vi "getSetting.vi"(8 "error in":errorcluster, 9 "Parameter":string="estimator_strategy", 10 "Array Parameter List":string[](array[string])=["izn3", "icomp"], 11 "Path":path=path "/home/ttsai/Documents/stash/ts_tcs_ofc/configData/pinv.esti") -> (0 "error out":errorcluster, 1 "Value":string)   [LabVIEW 2016]
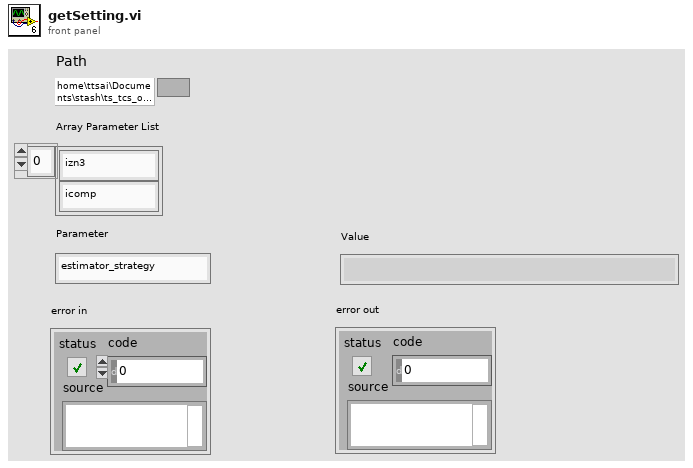
[diagram p1: front panel]
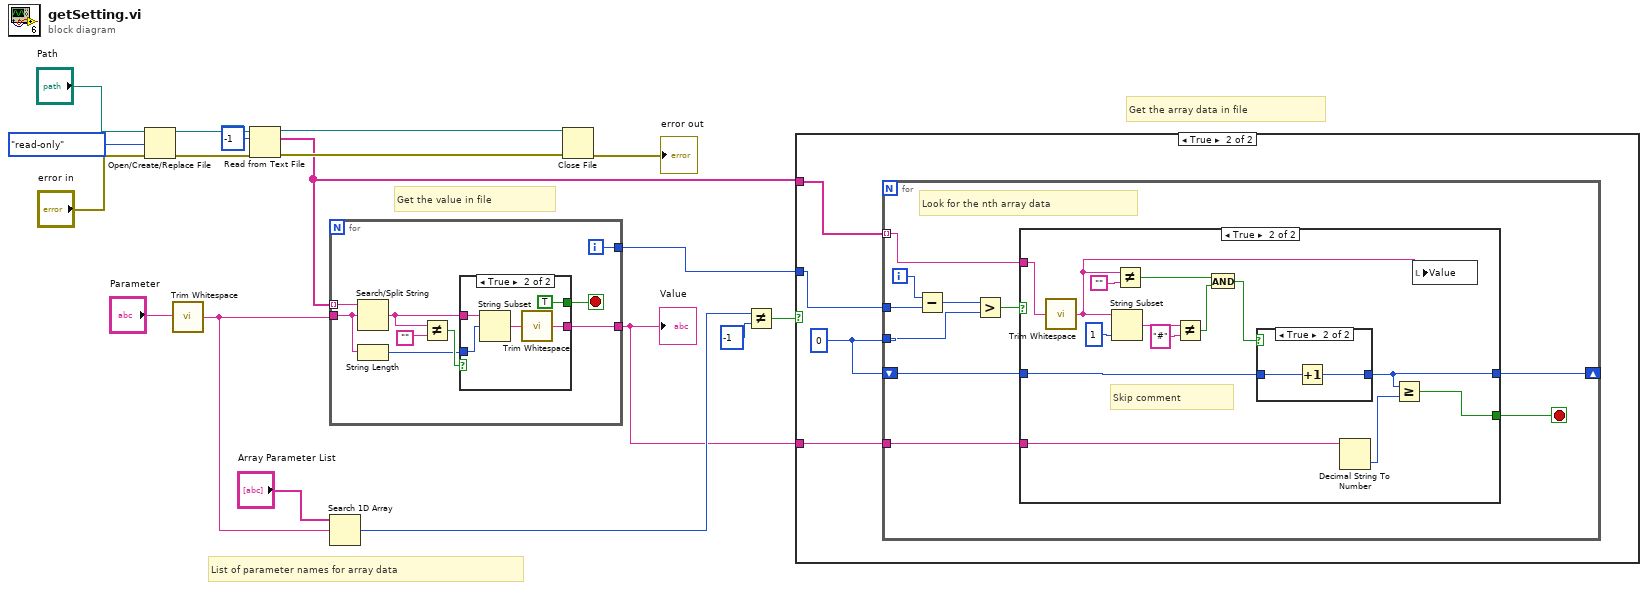
[diagram p0: block diagram]
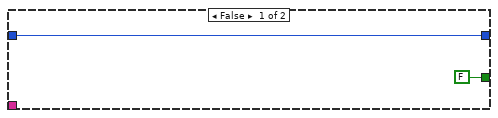
[diagram p3: hidden frame]
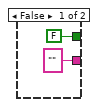
[diagram p5: hidden frame]
diagram:
  # "List of parameter names for array data"
  # "Get the array data in file"
  # "Get the value in file"
  n1 = Open/Create/Replace File(file path (use dialog)="Path", error in="error in", access (0:read/write)=enum16{"read/write", "read-only", "write-only"}."read-only") -> (refnum out=w15:refnum<file>, error out=w13:errorcluster)  [unwired: 3 in, 1 out]
  n2 = call <vilib>:"Trim Whitespace.vi"("string"="Parameter") -> ("trimmed string"=w7:string)  [unwired: 1 in]
  n3 = Read from Text File(file (use dialog)=w15, count=-1, error in=w13) -> (refnum out=w14:refnum<file>, text=w2:string[], error out=w12:errorcluster)  [unwired: 1 in, 1 out]
  n4 = for {
    tunnel: w2 -> [w20] mode=indexing
    tunnel: w7 -> [w23]
    tunnel: [w22] -> w1
    tunnel: [w21] -> w3
    i -> [w21]
    stop <- w26 stop-if-true
    n5 = Search/Split String(string=w20, search string/char (-)=w23) -> (match + rest of string=w25:string)  [unwired: 1 in, 2 out]
    n6 = String Length(string=w23) -> (length=w24:i32)
    n7 = Not Equal?(x=w25, y="") -> (x != y?=w27:bool)
    n8 = case shown="True" w27 {
      tunnel: [FALSE TRUE] -> w26
      tunnel: w25 -> [_ w33]
      tunnel: ["" w30] -> w22
      tunnel: w24 -> [_ w32]
      frame False {
      }
      frame True {
        n9 = String Subset(string=w33, offset (0)=w32) -> (substring=w31:string)  [unwired: 1 in]
        n10 = call <vilib>:"Trim Whitespace.vi"("string"=w31) -> ("trimmed string"=w30:string)  [unwired: 1 in]
      }
    }
  }
  "Value" <- w1
  n11 = Search 1D Array(1D array="Array Parameter List", element=w7) -> (index of element=w5:i32)  [unwired: 1 in]
  n12 = Close File(refnum=w14, error in=w12) -> (error out=→"error out":errorcluster)  [unwired: 1 out]
  n13 = Not Equal?(x=w5, y=-1) -> (x != y?=w6:bool)
  n14 = case shown="True" w6 {
    tunnel: w3 -> [_ w38]
    tunnel: w2 -> [_ w37]
    tunnel: w1 -> [_ w36]
    frame False {
    }
    frame True {
      w35 = 0 ("y")
      n15 = for {
        tunnel: w38 -> [w44]
        tunnel: w37 -> [w47] mode=indexing
        shift-right: [w40] -> _
        shift-left: w35 -> [w41]
        tunnel: w35 -> [w42]
        tunnel: w36 -> [w39]
        i -> [w45]
        stop <- w43 stop-if-true
        # "Look for the nth array data"
        n16 = Subtract(x=w45, y=w44) -> (x-y=w46:i32)
        n17 = Greater?(x=w46, y=w42) -> (0:w48:bool)
        n18 = case shown="True" w48 {
          tunnel: w47 -> [_ w64]
          tunnel: [FALSE w58] -> w43
          tunnel: w41 -> [w49 w62]
          tunnel: [w49 w61] -> w40
          tunnel: w39 -> [_ w60]
          frame False {
          }
          frame True {
            # "Skip comment"
            n19 = call <vilib>:"Trim Whitespace.vi"("string"=w64) -> ("trimmed string"=w51:string)  [unwired: 1 in]
            n20 = String Subset(string=w51, length (rest)=1 ("length (rest)")) -> (substring=w56:string)  [unwired: 1 in]
            n21 = Not Equal?(x=w51, y="") -> (x != y?=w54:bool)
            n22 = Not Equal?(x=w56, y="#") -> (x != y?=w53:bool)
            n23 = And(x=w54, y=w53) -> (x .and. y?=w52:bool)
            n24 = case shown="True" w52 {
              tunnel: w62 -> [w65 w67]
              tunnel: [w65 w66] -> w61
              frame False {
              }
              frame True {
                n25 = Increment(x=w67) -> (x+1=w66:i32)
              }
            }
            n26 = Decimal String To Number(string=w60) -> (number=w59:i32)  [unwired: 2 in, 1 out]
            n27 = Greater Or Equal?(x=w61, y=w59) -> (x >= y?=w58:bool)
            n28 = local write "Value"(w51) -> ()
          }
        }
      }
    }
  }
